vi "Send String Data.vi"(8 "Error In":errorcluster, 9 "timeout ms (25000)":i32, 10 "String Data":string, 11 "TCP In":refnum<k5>) -> (0 "Error Out":errorcluster, 3 "TCP Out":refnum<k5>)   [LabVIEW 2016, in "OPI.lvclass"]
doc: "Send string data prepend with its 4-byte size, formatted big endian."
uses:
  OPI.lvclass
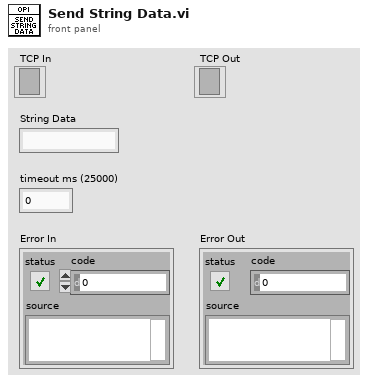
[diagram p1: front panel]
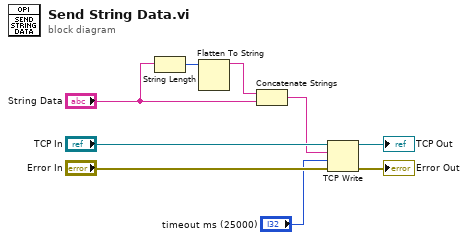
[diagram p0: block diagram]
diagram:
  n1 = String Length(string="String Data") -> (length=w4:i32)
  n2 = Flatten To String(anything=w4) -> (data string=w9:string)  [unwired: 3 in, 2 out]
  n3 = Concatenate Strings(w9, "String Data") -> (w6:string)
  n4 = TCP Write(connection ID="TCP In", data in=w6, error in (no error)="Error In", 9:"timeout ms (25000)") -> (connection ID out=→"TCP Out":refnum<k5>, error out=→"Error Out":errorcluster)  [unwired: 1 out]
